vi "DSF.Transceiver.UDP.Constants.Base Error Code.vi"() -> (3 "base error code":i32)   [LabVIEW 2017, in "DSF.Transceiver.UDP.lvlib" / "DSF.Transceiver.UDP.lvclass"]
uses:
  DSF.Transceiver.UDP.lvclass
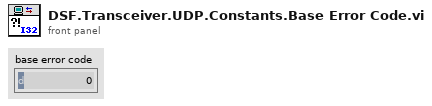
[diagram p1: front panel]
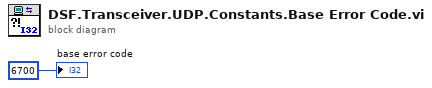
[diagram p0: block diagram]
diagram:
  "base error code" <- 6700 ("base error code")
